vi "ReferenceMove.vi"(8 "error in (no error)":errorcluster, 10 "AxisNumber":u8, 11 "CS++Motor in":refnum<class "CS++Motor.lvclass">) -> (0 "error out":errorcluster, 3 "CS++Motor out":refnum<class "CS++Motor.lvclass">)   [LabVIEW 2015, in "CS++Motor.lvlib" / "CS++Motor.lvclass"]
doc: "Starts a movement to the reference switch of this axis. Once the motor reaches the reference switch it should slowly move down from the switch and stop. Afterwards the internal step counter is set to zero. \n\nThe main purpose of this function is to calibrate the motor."
uses:
  CS++Motor.lvclass
  CS++Motor.lvclass/CS++Motor.ctl
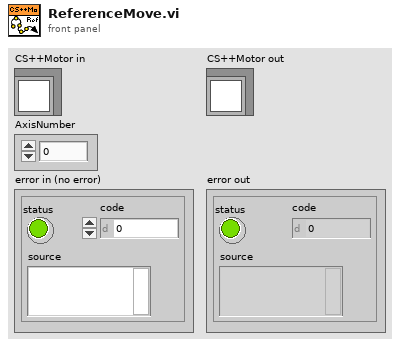
[diagram p1: front panel]
types:
  T1 = enum16{"NormalMovement", "ReferenceMovement", "StopMovement"}
  T2 = cluster{"Command":string, "AxisNumber":u8, "Data":variant}
  T3 = cluster{"MovementType":enum16{"NormalMovement", "ReferenceMovement", "StopMovement"}, "SetPosition":dbl, "Relative?":bool}
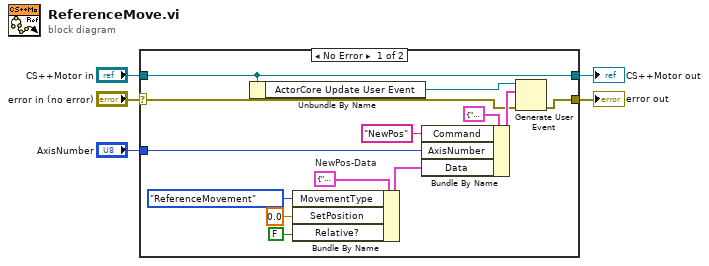
[diagram p0: block diagram]
diagram:
  n1 = case shown="No Error" "error in (no error)" {
    selector: "error in (no error)" -> [w10 w20]
    tunnel: [w15 w20] -> w4
    tunnel: [w9 w19] -> w5
    tunnel: "CS++Motor in" -> [w9 w19]
    tunnel: "AxisNumber" -> [w14 _]
    frame No Error {
      w12 = T3 {"MovementType"=enum."NormalMovement", "SetPosition"=0.0, "Relative?"=FALSE}  # NewPos-Data
      n2 = Unbundle By Name(w9) -> ("ActorCore Update User Event"=w8:refnum<user-event>)
      n3 = Bundle By Name(cluster=w12, "MovementType"=T1."ReferenceMovement", "SetPosition"=0.0, "Relative?"=FALSE) -> (w13:T3)
      n4 = Bundle By Name(cluster=T2 {"Command"="", "AxisNumber"=0, "Data"=variant} ("event data"), "Command"="NewPos", "AxisNumber"=w14, "Data"=w13) -> (w17:T2)
      n5 = Generate User Event(user event=w8, event data cluster=w17, error in=w10) -> (error out=w15:errorcluster)  [unwired: 1 in, 1 out]
    }
    frame Error {
    }
  }
  "error out" <- w4
  "CS++Motor out" <- w5
